vi "Sum Above Threshold.vi"(0 "Array":dbl[][](array[numeric]), 11 "Threshold":dbl) -> (8 "Sum Threshold":dbl)   [LabVIEW 2020]
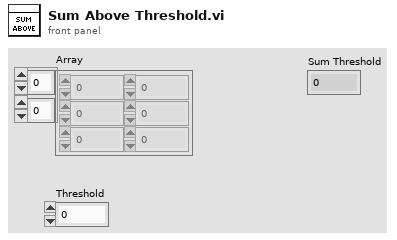
[diagram p1: front panel]
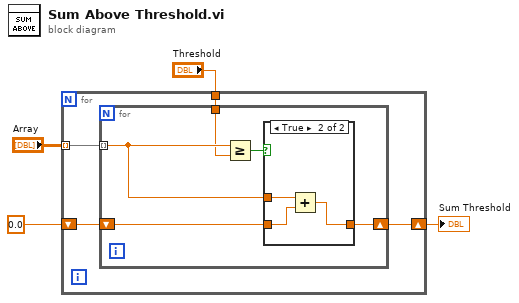
[diagram p0: block diagram]
diagram:
  n1 = for {
    tunnel: "Array" -> [w8] mode=indexing
    shift-right: [w6] -> w1
    shift-left: 0.0 -> [w7]
    tunnel: "Threshold" -> [w5]
    n2 = for {
      tunnel: w8 -> [w12] mode=indexing
      shift-right: [w10] -> w6
      shift-left: w7 -> [w11]
      tunnel: w5 -> [w9]
      n3 = Greater Or Equal?(x=w12, y=w9) -> (x >= y?=w13:bool)
      n4 = case shown="True" w13 {
        tunnel: w12 -> [_ w16]
        tunnel: w11 -> [w14 w17]
        tunnel: [w14 w15] -> w10
        frame False {
        }
        frame True {
          n5 = Add(x=w16, y=w17) -> (x+y=w15:dbl)
        }
      }
    }
  }
  "Sum Threshold" <- w1
